vi "FT_Get_Device_Info_List_64bit.vi"(0 "Number Of Devices":u32) -> (1 "FT_Status":u32(ring) items=["FT_OK", "FT_INVALID_HANDLE", "FT_DEVICE_NOT_FOUND", "FT_DEVICE_NOT_OPENED", "FT_IO_ERROR", "FT_INSUFFICIENT_RESOURCES", "FT_INVALID_PARAMETER", "FT_INVALID_BAUD_RATE", "FT_DEVICE_NOT_OPENED_FOR_ERASE", "FT_DEVICE_NOT_OPENED_FOR_WRITE", "FT_FAILED_TO_WRITE_DEVICE", "FT_EEPROM_READ_FAILED", "FT_EEPROM_WRITE_FAILED", "FT_EEPROM_ERASE_FAILED", "FT_EEPROM_NOT_PRESENT", "FT_EEPROM_NOT_PROGRAMMED", "FT_INVALID_ARGS", "FT_NOT_SUPPORTED", "FT_OTHER_ERROR"], 2 "Device Info List":T1(array[cluster]) {"FT_Handle" format="%.0x"; "LocID" format="%.0x"; "PID" format="%.0x"; "VID" format="%.0x"; "Type" items=["FT232B-FT245B", "FT8U232AM-FT8U245AM", "FT8U100AX", "UNKNOWN", "FT2232", "FT232R", "FT2232H", "FT4232H"]})   [LabVIEW 2018]
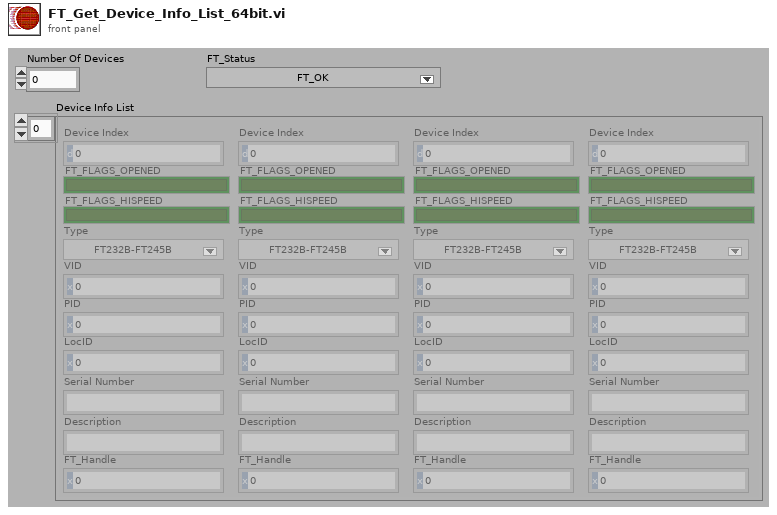
[diagram p1: front panel]
types:
  T1 = cluster{"Device Index":u32, "FT_FLAGS_OPENED":bool, "FT_FLAGS_HISPEED":bool, "Type":u32, "VID":u32, "PID":u32, "LocID":i32, "Serial Number":string, "Description":string, "FT_Handle":u32}[]
  T2 = cluster{"Device Index":u32, "FT_FLAGS_OPENED":bool, "FT_FLAGS_HISPEED":bool, "Type":u32, "VID":u32, "PID":u32, "LocID":i32, "Serial Number":string, "Description":string, "FT_Handle":u32}
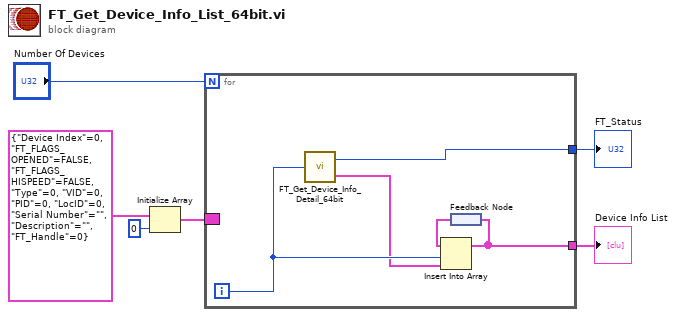
[diagram p0: block diagram]
diagram:
  n1 = Initialize Array(T2 {"Device Index"=0, "FT_FLAGS_OPENED"=FALSE, "FT_FLAGS_HISPEED"=FALSE, "Type"=0, "VID"=0, "PID"=0, "LocID"=0, "Serial Number"="", "Description"="", "FT_Handle"=0} ("Device Info Node"), 0 ("dimension size")) -> (w5:T1)
  n2 = for {
    N: "Number Of Devices" -> [_]
    tunnel: [w10] -> w2
    tunnel: [w8] -> w3
    border: w5 -> [_]
    i -> [w9]
    n3 = call "FT_Get_Device_Info_Detail_64bit.vi"("Device Index"=w9) -> ("FT_Status"=w8:u32, "Device Info Node"=w7:T2)
    n4 = feedback #1() -> (w11:T1)
    n5 = Insert Into Array(array=w11, index=w9, new element=w7) -> (w10:T1)
    n6 = feedback-in #1(w10) -> ()
  }
  "FT_Status" <- w3
  "Device Info List" <- w2
